vi "BRig_Host_dataRunState__clearData.vi"(9 "input_idx":i32[](array[numeric]), 10 "input_dataTS":u16[][](array[numeric]), 11 "input_dataPlot":u16[][](array[numeric])) -> (1 "output_idx":i32[](array[numeric]), 2 "output_dataTS":u16[][](array[numeric]), 3 "output_dataPlot":u16[][](array[numeric]))   [LabVIEW 2014]
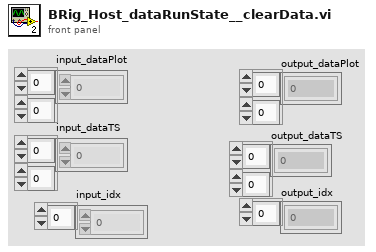
[diagram p1: front panel]
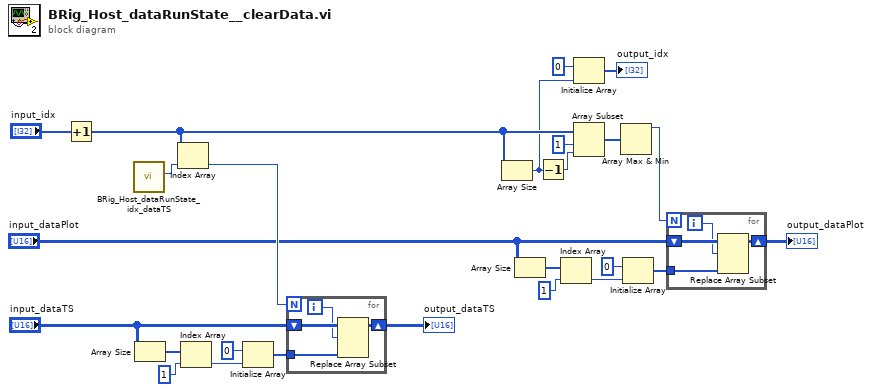
[diagram p0: block diagram]
diagram:
  n1 = Increment(x="input_idx") -> (x+1=w14:i32[])
  n2 = call "BRig_Host_dataRunState_idx_dataTS.vi"() -> ("output_idx_dataTS"=w25:i32)  [unwired: 11 in]
  n3 = Array Size(array="input_dataTS") -> (size(s)=w23:i32[])
  n4 = Index Array(array=w14, index=w25) -> (element=w18:i32)
  n5 = Index Array(array=w23, index=1) -> (element=w19:i32)
  n6 = Initialize Array(u16 0 ("element"), w19) -> (w17:u16[])
  n7 = for {
    N: w18 -> [_]
    shift-right: [w28] -> w16
    shift-left: "input_dataTS" -> [w29]
    tunnel: w17 -> [w26]
    i -> [w27]
    n8 = Replace Array Subset(array=w29, new element=w26, index (row)=w27) -> (w28:u16[][])  [unwired: 1 in]
  }
  "output_dataTS" <- w16
  n9 = Array Size(array=w14) -> (size(s)=w3:i32)
  n10 = Array Size(array="input_dataPlot") -> (size(s)=w11:i32[])
  n11 = Decrement(x=w3) -> (x-1=w13:i32)
  n12 = Index Array(array=w11, index=1) -> (element=w8:i32)
  n13 = Initialize Array(0 ("element"), w3) -> (→"output_idx":i32[])
  n14 = Array Subset(array=w14, index=1, length=w13) -> (w12:i32[])
  n15 = Array Max & Min(array=w12) -> (max value=w5:i32)  [unwired: 3 out]
  n16 = Initialize Array(u16 0 ("element"), w8) -> (w7:u16[])
  n17 = for {
    N: w5 -> [_]
    shift-right: [w32] -> w4
    shift-left: "input_dataPlot" -> [w33]
    tunnel: w7 -> [w30]
    i -> [w31]
    n18 = Replace Array Subset(array=w33, new element=w30, index (row)=w31) -> (w32:u16[][])  [unwired: 1 in]
  }
  "output_dataPlot" <- w4
